vi "Search_Table_SQL.vi"(7 "error in (no error)":errorcluster, 9 "Table name":string, 10 "Refnum in":T1) -> (0 "error out":errorcluster, 1 "Table List":string[](array[string]), 3 "Refnum out":T1)   [LabVIEW 2017]
uses:
  <vilib>/addons/database/Connection.llb/Conn ObjectReference.ctl
  <vilib>/regexp/Match Regular Expression.xnode
  <vilib>/addons/database/NI_Database_API.lvlib
panel:
  out "tables":string[](array[string])
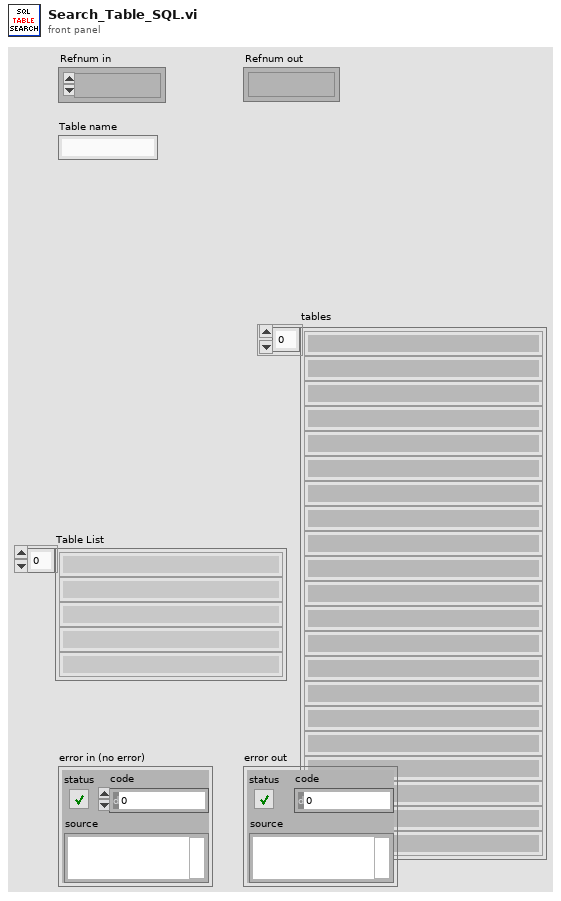
[diagram p1: front panel]
types:
  T1 = typedef "NI_Database_API.lvlib/Conn ObjectReference.ctl" = refnum<k1>
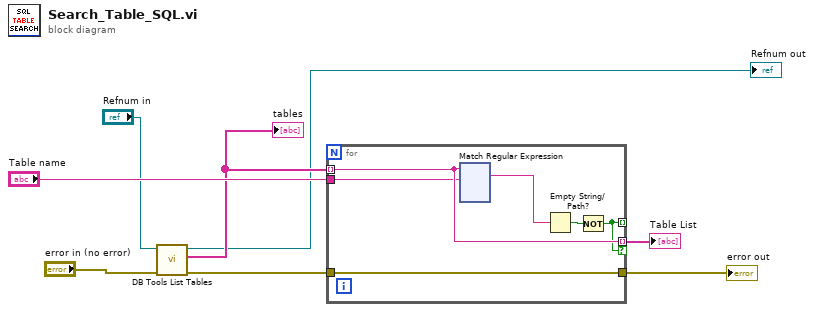
[diagram p0: block diagram]
diagram:
  n1 = call <vilib>:"DB Tools List Tables.vi"("error in (no error)"="error in (no error)", "connection reference"="Refnum in") -> ("error out"=w2:errorcluster, "tables"=w6:string[], "connection reference out"=→"Refnum out":T1)  [unwired: 3 in]
  "tables" <- w6
  n2 = for {
    tunnel: w6 -> [w13] mode=indexing
    tunnel: [w11] -> _ mode=indexing
    tunnel: [w13] -> w7 mode=indexing if=w11
    tunnel: "Table name" -> [w10]
    tunnel: [w9] -> w1
    tunnel: w2 -> [w9]
    n3 = xnode "Match Regular Expression"("input string"=w13, "regular expression"=w10) -> ("whole match"=w14:string)  [unwired: 4 in, 4 out]
    n4 = Empty String/Path?(string/path=w14) -> (empty?=w12:bool)
    n5 = Not(x=w12) -> (.not. x?=w11:bool)
  }
  "Table List" <- w7
  "error out" <- w1
